vi "FGV-Funktionstasten.vi"(0 "Referenz":refnum<vi>, 1 "Samplepoint":u16, 2 "Herkunft":string="---", 5 "Funktionstasten":T4, 7 "Zeit":sgl, 9 "Zustand":T2, 11 "Fehler (FALSE)":bool, 12 "Aktion":T3=enum."Lesen") -> (3 "Samplepoint":u16, 4 "EXTERN Umschalten":bool, 6 "Zustand Herkunft AK?":bool, 8 "Zeit Zustands Anwahl":timestamp, 10 "ausgewählte Funktion":T2, 13 "Busy":bool, 14 "Betriebsart":T1, 15 "Fehler steht an":bool)   [LabVIEW 2020, in "Funktionstasten.lvlib"]
doc: "Führt die durch den Enum \"Aktion\" geforderte Aktion aus, indem über eine Referenz auf den Cluster \"Funktionstasten\" die Beschriftungen und Tastenfarben manipuliert werden. Der Eingang \"Funktionstasten\" ist neben der Referenz notwendig, um bei einer Ereignis-gesteuerten Tastenreaktion eine gedrückte Taste zui erkennen, die Latch-Verhalten hat.\n\nDie funktionale globale Variable (FGV) speichert den aktuellen Zustand der Tasten und des aktuellen Fehlerstatus. Die FGV kann von Sub-VIs und fremden VIs aufgerufen werden. Außer dem Eingang \"Aktion\" sind alle Eingänge sind nur \"empfohlen\" und nicht immer \"erforderlich\", -abhängig von der Aktion:\n\nInitialisieren:\nSpeichert eine Referenz auf den Cluster\"Funktionstasten\" und macht alle Tasten vorläufig nicht anwählbar. Erst nach dem vollständigen Hochlauf sollten die Tasten durch die Aktion \"Zustand setzen\" in einem definierten Zustand aktiviert werden. Dabei werden die Beschriftungen der Tasten vom Enum \"Zustand\" übernommen und gespeichert.\nNur Eingang \"Referenz\" erforderlich.\n\nZustand setzen:\nÄndert den Tastenzustand programmgesteuert auf den am Eingang \"Zustand\" anliegenden Wert.\nNur Eingang \"Zustand\" erforderlich.\n\nTaste gedrückt:\nMarkiert die gedrückte Taste entsprechend dem gespeicherten Fehlerzustand und liefert die ausgewählte Funktion zur Steuerung eines Zustandsautomaten.\nNur Eingang \"Funktionstasten\" erforderlich.\n\nFehler speichern:\nÜbernimmt den Eingang \"Fehler\" und speichert ihn als \"Fehler steht an\".\nNur Eingang \"Fehler\" erforderlich.\n\nZustand lesen:\nLiefert die durch den letzten Tastendruck ausgewählte, gespeicherte Funktion und den Fehlerstatus.\nKeine Eingänge notwendig.\n\nManuell:\nAktiviert den Bedienerzugriff auf die Tasten für Handbetrieb.\nKeine Eingänge notwendig.\n\nRemote:\nDie Tasten sind nur mehr über die Aktion \"Zustand setzen\" anwählbar, die aktuelle Taste und der Fehlerzustand werden aber angezeigt.\nKeine Eingänge notwendig."
uses:
  Funktionstasten.lvlib
  Funktionstasten.ctl
  Funktionstasten-Aktion.ctl
  Zustaende.ctl
  Betriebsart.ctl
  Freigabe Aktionen.ctl
  Sprachverwaltung/FGV Aktion Tabelle zerlegen.ctl
  Aktionen Zustaende Loggen.ctl
  Seiten/Anlagenuebersicht/VisBx Anzeige/Aktion FGV Ventile manuell schalten Crio.ctl
  PNS/Aktionen FGV Grenzwerte.ctl
  SysLog/SysLog Interface.ctl
  PNS/PNS.lvlib
  Sprachverwaltung/Sprachverwaltung.lvlib
  Amium PNS/Amium PNS.lvlib
  SysLog/SysLog.lvlib
  <vilib>/Utility/Data Type/NI_Data Type.lvlib
  Seiten/Anlagenuebersicht/VisBx Anzeige/Anlagenuebersicht.lvlib
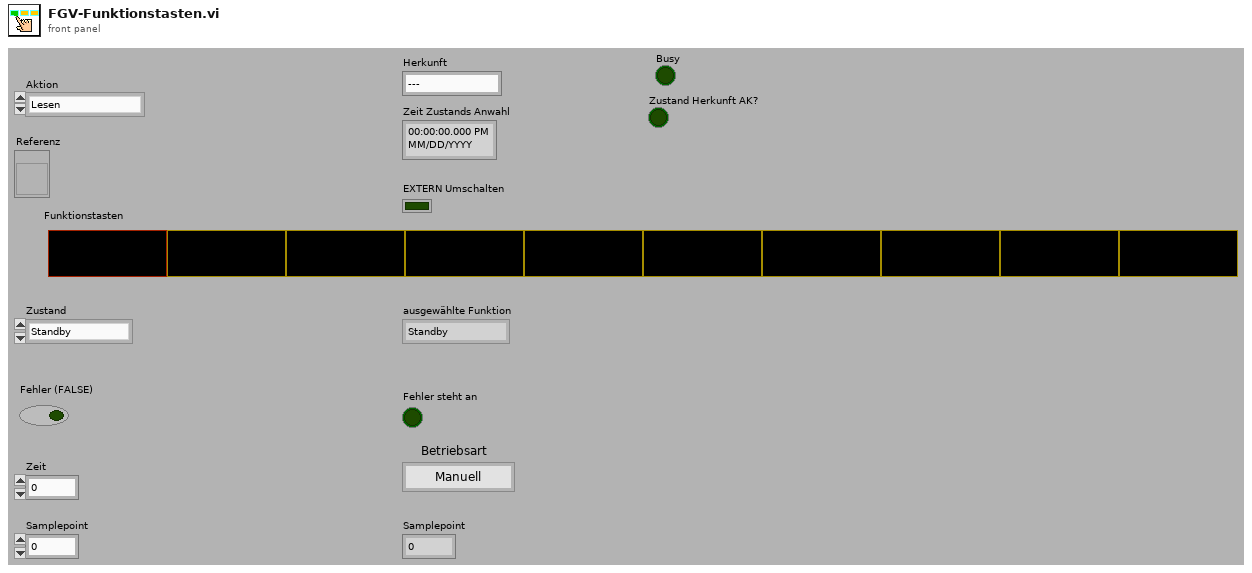
[diagram p1: front panel]
types:
  T1 = typedef "Funktionstasten.lvlib/Betriebsart.ctl" = enum16{"Manuell", "Remote", "Bitparallel"}
  T2 = typedef "Funktionstasten.lvlib/Zustaende.ctl" = enum16{"Standby", "Pause", "Eco", "Messen", "Kalibrieren", "Spülen Filter", "Spülen Leitung", "Umgebungsluft", "0-Gas", "Cal-Gas", "CG zu PNS", "-------------", "Init 1", "Init 2", "Init 3", "Init 4", "Messen vorbereiten", "Messen durchführen", "Exit"}
  T3 = typedef "Funktionstasten.lvlib/Funktionstasten-Aktion.ctl" = enum16{"Initialisieren", "Zustand setzen", "Taste gedrückt", "Fehler speichern", "Lesen", "Manuell", "Remote", "Bitparallel", "Samplepoint", "Zeit Prüfen", "reset Umschalten"}
  T4 = typedef "Funktionstasten.lvlib/Funktionstasten.ctl" = cluster{"Taste 1":bool, "Taste 2":bool, "Taste 3":bool, "Taste 4":bool, "Taste 5":bool, "Taste 6":bool, "Taste 7":bool, "Taste 11":bool, "Taste 9":bool, "Taste 10":bool}
  T5 = typedef "Funktionstasten.lvlib/Freigabe Aktionen.ctl" = enum16{"prüfen", "Freigabe?", "lesen"}
  T6 = typedef "Sprachverwaltung.lvlib/FGV Aktion Tabelle zerlegen.ctl" = enum16{"laden", "vereinzeln", "speichern"}
  T7 = typedef "Anlagenuebersicht.lvlib/Aktion FGV Ventile manuell schalten Crio.ctl" = enum16{"lesen", "Ventile schalten", "Testbetrieb aktiv", "Testbetrieb inaktiv", "Anzeige Ventilstellung"}
  T8 = typedef "Funktionstasten.lvlib/Aktionen Zustaende Loggen.ctl" = enum16{"lesen", "schreiben", "löschen", "init"}
  T9 = typedef "PNS.lvlib/Aktionen FGV Grenzwerte.ctl" = enum16{"lesen", "Grenzw. schreiben", "Anweisungscode", "IP-Adresse", "laden", "speichern", "Anweisungscode vorgeben"}
  T10 = typedef "SysLog.lvlib/SysLog Interface.ctl" = cluster{"FehlermeldungsCode":i32, "ErfolgsmeldungsCode":i32, "ParameterListenString":string, "Anzeige":bool, "SysLogIcon":enum16{"OK", "Warnung", "Fehler"}, "intern":bool}
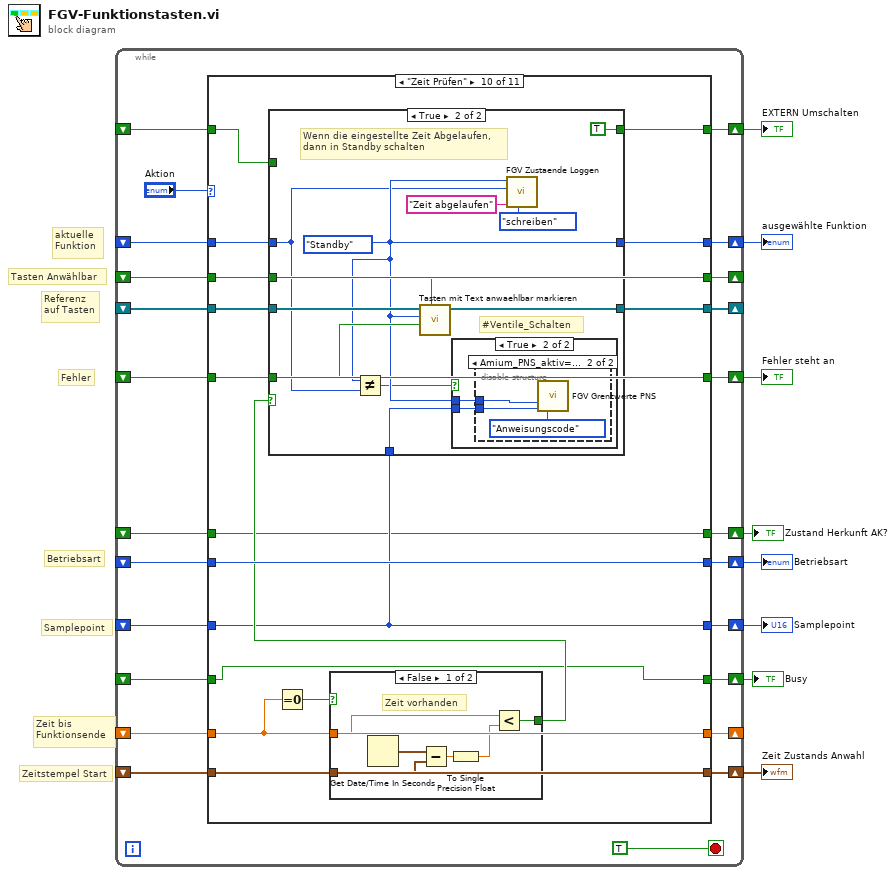
[diagram p0: block diagram]
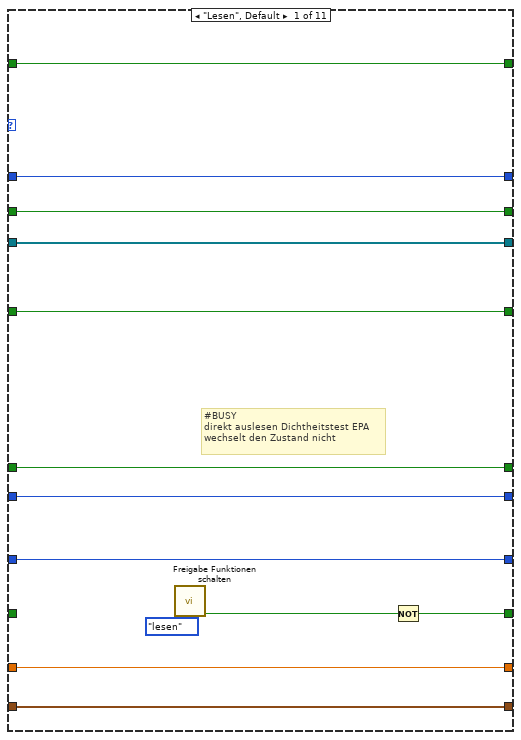
[diagram p2: hidden frame]
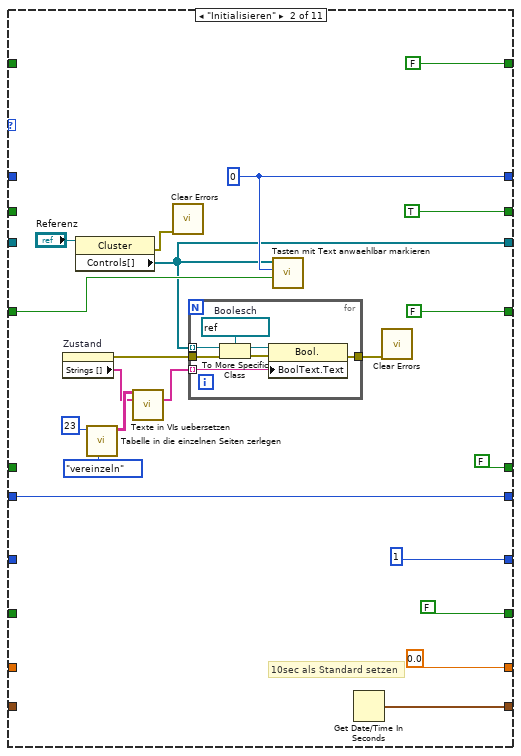
[diagram p3: hidden frame]
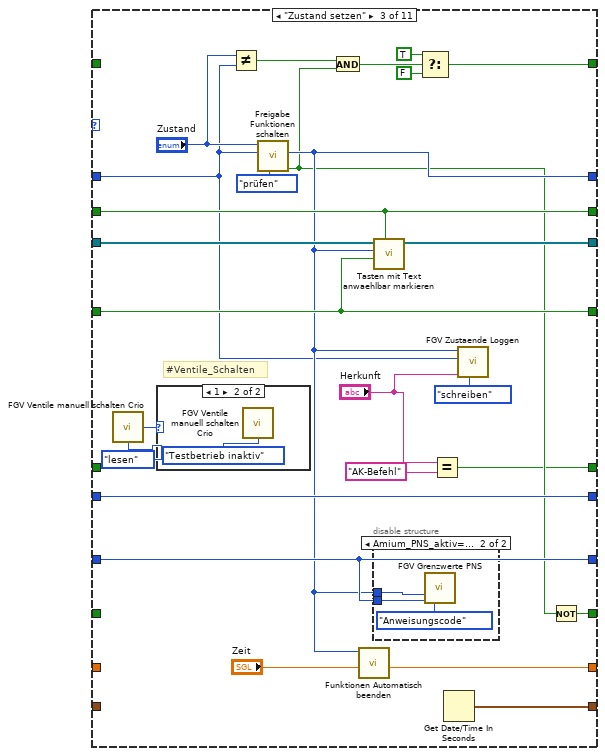
[diagram p4: hidden frame]
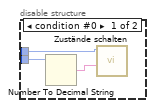
[diagram p6: hidden frame]
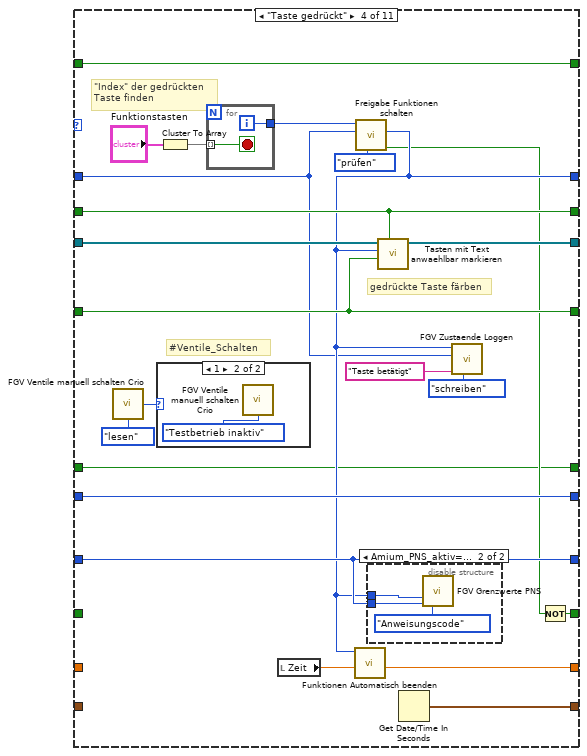
[diagram p7: hidden frame]
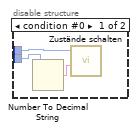
[diagram p9: hidden frame]
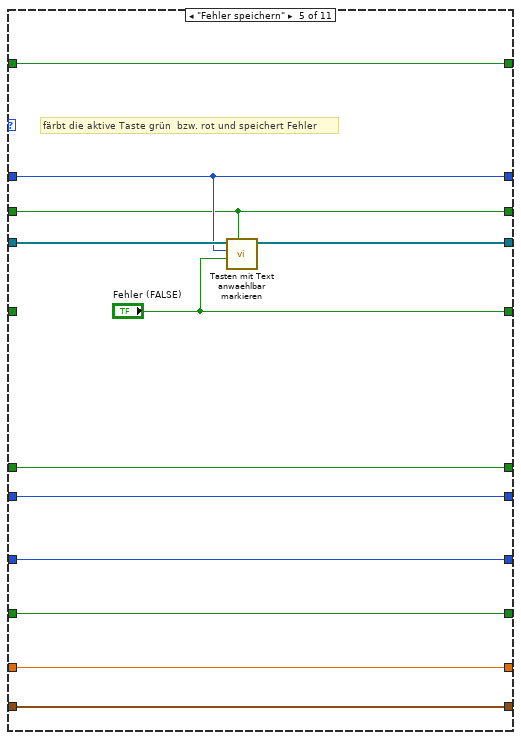
[diagram p10: hidden frame]
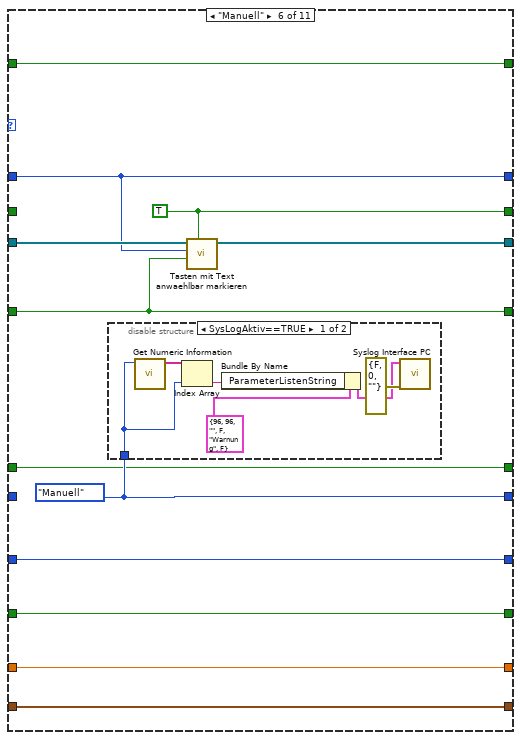
[diagram p11: hidden frame]
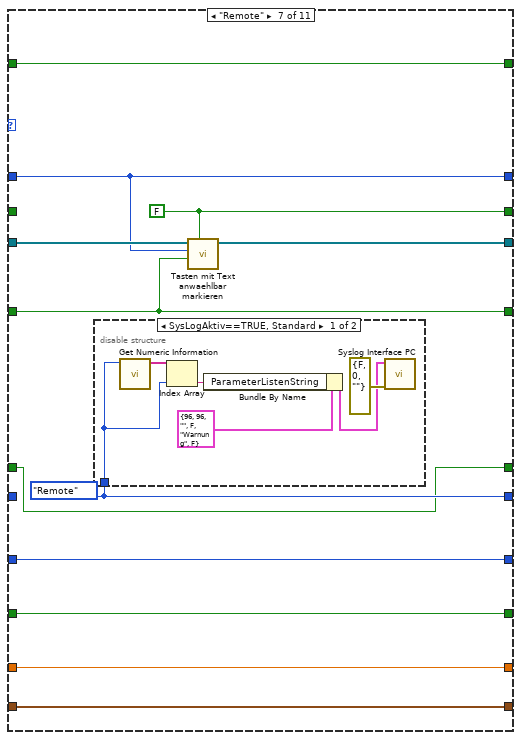
[diagram p13: hidden frame]
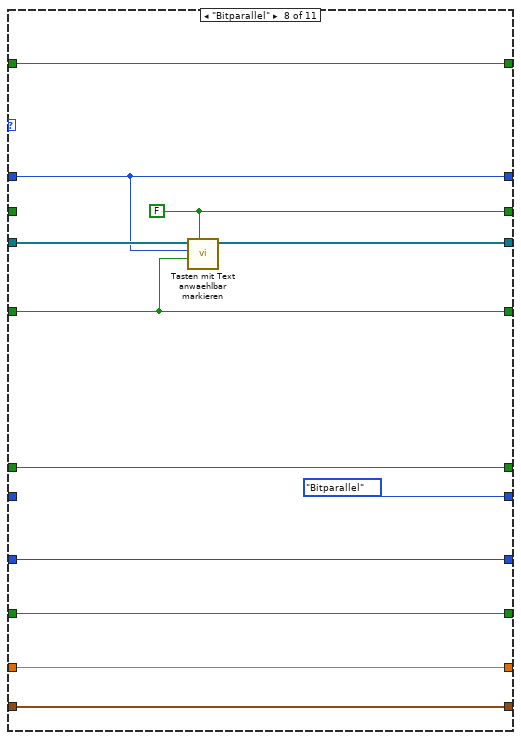
[diagram p15: hidden frame]
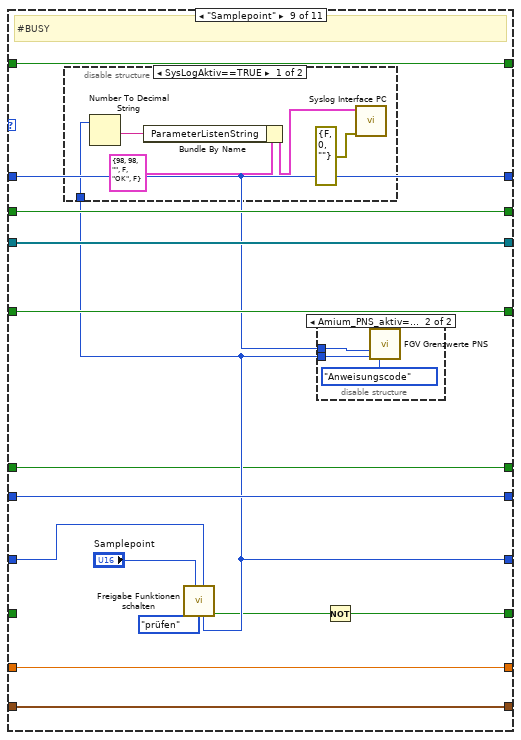
[diagram p16: hidden frame]
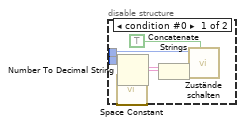
[diagram p18: hidden frame]
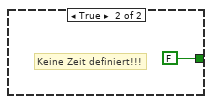
[diagram p19: hidden frame]
diagram:
  # "Zeitstempel Start"
  # "Samplepoint"
  # "Betriebsart"
  # "Tasten Anwählbar"
  # "Zeit bis \nFunktionsende"
  # "Fehler"
  # "aktuelle\nFunktion"
  # "Referenz\nauf Tasten"
  n1 = while {
    shift-right: [w18] -> w5
    shift-left: _ -> [w32]
    shift-right: [w29] -> _
    shift-left: _ -> [w28]
    shift-right: [w27] -> w8
    shift-left: _ -> [w21]
    shift-right: [w26] -> _
    shift-left: _ -> [w25]
    shift-right: [w24] -> _
    shift-left: _ -> [w23]
    shift-right: [w22] -> w7
    shift-left: _ -> [w20]
    shift-right: [w17] -> w6
    shift-left: _ -> [w19]
    shift-right: [w16] -> w3
    shift-left: _ -> [w15]
    shift-right: [w14] -> w4
    shift-left: _ -> [w13]
    shift-right: [w12] -> w2
    shift-left: _ -> [w11]
    shift-right: [w10] -> w1
    shift-left: _ -> [w9]
    stop <- TRUE stop-if-true
    n2 = case shown="\"Zeit Prüfen\"" "Aktion" {
      tunnel: w28 -> [w44 _ w99 w127 w149 w161 w177 w195 w210 w242 w279]
      tunnel: [w45 w63 w82 w114 w146 w159 w175 w193 w206 w240 w281] -> w18
      tunnel: w32 -> [w45 _ w81 w113 w146 w159 w175 w193 w206 w237 w281]
      tunnel: [w44 w62 w98 w126 w148 w160 w178 w196 w210 w239 w279] -> w29
      tunnel: w25 -> [w42 _ _ _ w150 w162 w180 w198 w211 w234 w276]
      tunnel: w21 -> [w43 w64 w96 w124 _ w157 w176 w194 w213 w241 w283]
      tunnel: [w43 FALSE ("Fehler (FALSE)") w96 w124 "Fehler (FALSE)" w157 w176 w194 w213 w241 w283] -> w27
      tunnel: [w42 sgl 0.0 w92 w121 w150 w162 w180 w198 w211 w234 w276] -> w26
      tunnel: [w41 TRUE ("Fehler (FALSE)") w97 w125 w145 w158 w179 w197 w209 w238 w280] -> w24
      tunnel: w23 -> [w41 _ w97 w125 w145 _ _ _ w209 w238 w280]
      tunnel: [w40 w60 w95 w123 w144 w153 w171 Betriebsart."Bitparallel" ("Betriebsart") w212 w243 w278] -> w22
      tunnel: w20 -> [w40 w60 w95 w123 w144 _ _ _ w212 w243 w278]
      tunnel: [w39 u16 1 ("Samplepoint") w84 w116 w143 w156 w174 w191 w202 w230 w277] -> w17
      tunnel: w19 -> [w39 _ w84 w116 w143 w156 w174 w191 w203 w230 w277]
      tunnel: [w38 w57 w94 w122 w142 w155 w173 w190 w208 w233 w275] -> w16
      tunnel: w15 -> [w38 _ _ _ w142 w155 w173 w190 w208 w233 w275]
      tunnel: [w37 FALSE w85 w117 w141 w154 w172 w189 w207 w231 FALSE] -> w14
      tunnel: w13 -> [w37 _ _ w117 w141 w154 w172 w189 w207 w232 _]
      tunnel: [w34 FALSE w80 w111 w140 w152 w170 w188 w200 w229 w274] -> w12
      tunnel: w11 -> [_ _ _ _ w140 w152 w170 w188 _ w229 w274]
      tunnel: [w36 FALSE w76 w109 w139 w151 w169 w187 w199 w228 w273] -> w10
      tunnel: w9 -> [w36 _ _ w109 w139 w151 w169 w187 w199 w228 w273]
      frame "Lesen", Default {
        # "#BUSY\ndirekt auslesen Dichtheitstest EPA \nwechselt den Zustand nicht"
        n3 = call "Freigabe Funktionen schalten.vi"("Aktionen"=Freigabe_Aktionen."lesen") -> ("Freigabe?"=w35:bool)  [unwired: 8 in, 2 out]
        n4 = Not(x=w35) -> (.not. x?=w34:bool)
      }
      frame "Initialisieren" {
        w63 = 0 ("Zustand")
        # "10sec als Standard setzen"
        n5 = property on="Zustand" class="Enum (strikt)"() -> (error out=w54:errorcluster, "Strings []"=w50:string[])  [unwired: 2 in, 1 out]
        n6 = property class="Cluster"(reference="Referenz") -> (error out=w55:errorcluster, "Controls[]"=w62:refnum<vi>[])  [unwired: 1 in, 1 out]
        n7 = call "Tabelle in die einzelnen Seiten zerlegen.vi"("Aktion"=FGV_Aktion_Tabelle_zerlegen."vereinzeln", "Index (Seite)"=23) -> ("Sprachliste"=w51:string[][])  [unwired: 7 in, 2 out]
        n8 = call "Texte in VIs uebersetzen.vi"("Sprachliste"=w51, "String-Array zum Übersetzen"=w50) -> ("String-Array zum Übersetzen"=w49:string[])  [unwired: 9 in, 4 out]
        n9 = call <vilib>:"Clear Errors.vi"("error in (no error)"=w55) -> ()  [unwired: 5 in, 2 out]
        n10 = for {
          tunnel: w49 -> [w70] mode=indexing
          tunnel: w62 -> [w72] mode=indexing
          tunnel: w54 -> [w68]
          tunnel: [w67] -> w53
          w73 = refnum<vi> refnum  # Boolesch
          n11 = To More Specific Class(target class=w73, reference=w72, error in=w68) -> (specific class reference=w71:refnum<vi>, error out=w69:errorcluster)
          n12 = property class="Bool."(reference=w71, error in=w69, "BoolText.Text"=w70) -> (error out=w67:errorcluster)  [unwired: 1 out]
        }
        n13 = call "Tasten mit Text anwaehlbar markieren.vi"("Fehler"=w64, "Tastennummer"=w63, "Tastenreferenzen"=w62) -> ()  [unwired: 2 in, 7 out]
        n14 = Get Date/Time In Seconds() -> (seconds since 1Jan1904=w57:timestamp)
        n15 = call <vilib>:"Clear Errors.vi"("error in (no error)"=w53) -> ()  [unwired: 5 in, 2 out]
      }
      frame "Zustand setzen" {
        # "#Ventile_Schalten"
        n16 = call "FGV Ventile manuell schalten Crio.vi"("Aktion"=Aktion_FGV_Ventile_manuell_schalten_Crio."lesen") -> ("Betrieb"=w75:u16)  [unwired: 11 in, 3 out]
        n17 = case shown="1" w75 {
          frame 0, Default {
          }
          frame 1 {
            n18 = call "FGV Ventile manuell schalten Crio.vi"("Aktion"=Aktion_FGV_Ventile_manuell_schalten_Crio."Testbetrieb inaktiv") -> ()  [unwired: 11 in, 4 out]
          }
        }
        n19 = Not Equal?(x="Zustand", y=w81) -> (x != y?=w89:bool)
        n20 = call "Freigabe Funktionen schalten.vi"("Aktionen"=Freigabe_Aktionen."prüfen", "Zustand ALT"=w81, "Zustand NEU"="Zustand") -> ("Freigabe?"=w79:bool, "Zustand"=w82:T2)  [unwired: 6 in, 1 out]
        n21 = And(x=w89, y=w79) -> (x .and. y?=w88:bool)
        n22 = call "Funktionen Automatisch beenden.vi"("Zeit"="Zeit", "ausgewählte Funktion"=w82) -> ("Zeit"=w92:sgl)  [unwired: 9 in]
        n23 = call "Tasten mit Text anwaehlbar markieren.vi"("Anwählbar"=w97, "Fehler"=w96, "Tastennummer"=w82, "Tastenreferenzen"=w99) -> ("Tastenreferenzen (Kopie)"=w98:refnum<vi>[])  [unwired: 2 in, 5 out]
        n24 = disable-structure shown="Amium_PNS_aktiv==FALSE" {
          disable-tunnel: w84 -> [w101 w105]
          disable-tunnel: w82 -> [w103 w104]
          frame condition #0 {
            n25 = Number To Decimal String(number=w101) -> (decimal integer string=w102:string)  [unwired: 1 in]
            n26 = call "Zustände schalten.vi"("Samplepoint 2"=w102, "Zustand"=w103) -> ()  [unwired: 9 in, 1 out]
          }
          frame condition #1 (active) {
            n27 = call "FGV Grenzwerte PNS.vi"("Zustand"=w104, "Samplepoint"=w105, "Aktionen FGV Grenzwerte"=Aktionen_FGV_Grenzwerte."Anweisungscode") -> ()  [unwired: 10 in, 3 out]
          }
        }
        n28 = Select(t=TRUE, s=w88, f=FALSE) -> (s? t:f=w85:bool)
        n29 = Equal?(x="Herkunft", y="AK-Befehl" ("Herkunft")) -> (x = y?=w76:bool)
        n30 = Get Date/Time In Seconds() -> (seconds since 1Jan1904=w94:timestamp)
        n31 = call "FGV Zustaende Loggen.vi"("Aktionen Zustände Loggen"=Aktionen_Zustaende_Loggen."schreiben", "Herkunft"="Herkunft", "Zustand ALT"=w81, "Zustand NEU"=w82) -> ()  [unwired: 6 in, 2 out]
        n32 = Not(x=w79) -> (.not. x?=w80:bool)
      }
      frame "Taste gedrückt" {
        # "#Ventile_Schalten"
        # "gedrückte Taste färben"
        # "\"Index\" der gedrückten\nTaste finden"
        n33 = call "FGV Ventile manuell schalten Crio.vi"("Aktion"=Aktion_FGV_Ventile_manuell_schalten_Crio."lesen") -> ("Betrieb"=w107:u16)  [unwired: 11 in, 3 out]
        n34 = case shown="1" w107 {
          frame 0, Default {
          }
          frame 1 {
            n35 = call "FGV Ventile manuell schalten Crio.vi"("Aktion"=Aktion_FGV_Ventile_manuell_schalten_Crio."Testbetrieb inaktiv") -> ()  [unwired: 11 in, 4 out]
          }
        }
        n36 = Cluster To Array(cluster="Funktionstasten") -> (array=w129:bool[])
        n37 = for {
          tunnel: w129 -> [w137] mode=indexing
          tunnel: [w138] -> w119
          i -> [w138]
          stop <- w137 stop-if-true
        }
        n38 = local read "Zeit"() -> (w118:sgl)
        n39 = call "Freigabe Funktionen schalten.vi"("Aktionen"=Freigabe_Aktionen."prüfen", "Zustand ALT"=w113, "Zustand NEU"=w119) -> ("Freigabe?"=w110:bool, "Zustand"=w114:T2)  [unwired: 6 in, 1 out]
        n40 = call "Funktionen Automatisch beenden.vi"("Zeit"=w118, "ausgewählte Funktion"=w114) -> ("Zeit"=w121:sgl)  [unwired: 9 in]
        n41 = disable-structure shown="Amium_PNS_aktiv==FALSE" {
          disable-tunnel: w116 -> [w132 w135]
          disable-tunnel: w114 -> [w133 w134]
          frame condition #0 {
            n42 = Number To Decimal String(number=w132) -> (decimal integer string=w131:string)  [unwired: 1 in]
            n43 = call "Zustände schalten.vi"("Samplepoint 2"=w131, "Zustand"=w133) -> ()  [unwired: 9 in, 1 out]
          }
          frame condition #1 (active) {
            n44 = call "FGV Grenzwerte PNS.vi"("Zustand"=w134, "Samplepoint"=w135, "Aktionen FGV Grenzwerte"=Aktionen_FGV_Grenzwerte."Anweisungscode") -> ()  [unwired: 10 in, 3 out]
          }
        }
        n45 = call "Tasten mit Text anwaehlbar markieren.vi"("Anwählbar"=w125, "Fehler"=w124, "Tastennummer"=w114, "Tastenreferenzen"=w127) -> ("Tastenreferenzen (Kopie)"=w126:refnum<vi>[])  [unwired: 1 in, 6 out]
        n46 = Get Date/Time In Seconds() -> (seconds since 1Jan1904=w122:timestamp)
        n47 = call "FGV Zustaende Loggen.vi"("Aktionen Zustände Loggen"=Aktionen_Zustaende_Loggen."schreiben", "Herkunft"="Taste betätigt", "Zustand ALT"=w113, "Zustand NEU"=w114) -> ()  [unwired: 6 in, 2 out]
        n48 = Not(x=w110) -> (.not. x?=w111:bool)
      }
      frame "Fehler speichern" {
        # "färbt die aktive Taste grün  bzw. rot und speichert Fehler"
        n49 = call "Tasten mit Text anwaehlbar markieren.vi"("Anwählbar"=w145, "Fehler"="Fehler (FALSE)", "Tastennummer"=w146, "Tastenreferenzen"=w149) -> ("Tastenreferenzen (Kopie)"=w148:refnum<vi>[])  [unwired: 1 in, 6 out]
      }
      frame "Manuell" {
        w153 = Betriebsart."Manuell" ("Betriebsart")
        w158 = TRUE ("Anwählbar")
        n50 = disable-structure shown="SysLogAktiv==TRUE" {
          disable-tunnel: w153 -> [w166 _]
          frame condition #0 (active) {
            n51 = call <vilib>:"Get Numeric Information.vi"("variant"=w166) -> ("enum names"=w167:string[])  [unwired: 7 in, 3 out]
            n52 = Index Array(array=w167, index=w166) -> (element=w163:string)
            n53 = Bundle By Name(cluster=T10 {"FehlermeldungsCode"=96, "ErfolgsmeldungsCode"=96, "ParameterListenString"="", "Anzeige"=FALSE, "SysLogIcon"=enum."Warnung", "intern"=FALSE} ("Cluster (in)"), "ParameterListenString"=w163) -> (w164:T10)
            n54 = call "Syslog Interface PC.vi"("Fehler (in)"=errorcluster {"status"=FALSE, "code"=0, "source"=""}, "Cluster (in)"=w164) -> ()  [unwired: 9 in, 1 out]
          }
          frame condition #1 {
          }
        }
        n55 = call "Tasten mit Text anwaehlbar markieren.vi"("Anwählbar"=w158, "Fehler"=w157, "Tastennummer"=w159, "Tastenreferenzen"=w161) -> ("Tastenreferenzen (Kopie)"=w160:refnum<vi>[])  [unwired: 1 in, 6 out]
      }
      frame "Remote" {
        w171 = Betriebsart."Remote" ("Betriebsart")
        w179 = FALSE ("Anwählbar")
        n56 = disable-structure shown="SysLogAktiv==TRUE, Standard" {
          disable-tunnel: w171 -> [w184 _]
          frame condition #0 (active) {
            n57 = call <vilib>:"Get Numeric Information.vi"("variant"=w184) -> ("enum names"=w185:string[])  [unwired: 7 in, 3 out]
            n58 = Index Array(array=w185, index=w184) -> (element=w181:string)
            n59 = Bundle By Name(cluster=T10 {"FehlermeldungsCode"=96, "ErfolgsmeldungsCode"=96, "ParameterListenString"="", "Anzeige"=FALSE, "SysLogIcon"=enum."Warnung", "intern"=FALSE} ("Cluster (in)"), "ParameterListenString"=w181) -> (w182:T10)
            n60 = call "Syslog Interface PC.vi"("Fehler (in)"=errorcluster {"status"=FALSE, "code"=0, "source"=""}, "Cluster (in)"=w182) -> ()  [unwired: 9 in, 1 out]
          }
          frame condition #1 {
          }
        }
        n61 = call "Tasten mit Text anwaehlbar markieren.vi"("Anwählbar"=w179, "Fehler"=w176, "Tastennummer"=w175, "Tastenreferenzen"=w177) -> ("Tastenreferenzen (Kopie)"=w178:refnum<vi>[])  [unwired: 1 in, 6 out]
      }
      frame "Bitparallel" {
        w197 = FALSE ("Anwählbar")
        n62 = call "Tasten mit Text anwaehlbar markieren.vi"("Anwählbar"=w197, "Fehler"=w194, "Tastennummer"=w193, "Tastenreferenzen"=w195) -> ("Tastenreferenzen (Kopie)"=w196:refnum<vi>[])  [unwired: 1 in, 6 out]
      }
      frame "Samplepoint" {
        # "#BUSY"
        n63 = call "Freigabe Funktionen schalten.vi"("Samplepoint ALT"=w203, "Aktionen"=Freigabe_Aktionen."prüfen", "Samplepoint NEU"="Samplepoint") -> ("Freigabe?"=w201:bool, "Samplepoint"=w202:u16)  [unwired: 6 in, 1 out]
        n64 = disable-structure shown="SysLogAktiv==TRUE" {
          disable-tunnel: w202 -> [w217 _]
          frame condition #0 (active) {
            n65 = Number To Decimal String(number=w217) -> (decimal integer string=w214:string)  [unwired: 1 in]
            n66 = Bundle By Name(cluster=T10 {"FehlermeldungsCode"=98, "ErfolgsmeldungsCode"=98, "ParameterListenString"="", "Anzeige"=FALSE, "SysLogIcon"=enum."OK", "intern"=FALSE} ("Cluster (in)"), "ParameterListenString"=w214) -> (w215:T10)
            n67 = call "Syslog Interface PC.vi"("Fehler (in)"=errorcluster {"status"=FALSE, "code"=0, "source"=""}, "Cluster (in)"=w215) -> ()  [unwired: 9 in, 1 out]
          }
          frame condition #1 {
          }
        }
        n68 = disable-structure shown="Amium_PNS_aktiv==FALSE, Standard" {
          disable-tunnel: w206 -> [w224 w226]
          disable-tunnel: w202 -> [w221 w225]
          frame condition #0 {
            n69 = call <vilib>:"Space Constant.vi"() -> ("String"=w219:string)
            n70 = Number To Decimal String(number=w221) -> (decimal integer string=w222:string)  [unwired: 1 in]
            n71 = Concatenate Strings(w219, w222) -> (w220:string)
            n72 = call "Zustände schalten.vi"("Samplepoint setzen"=TRUE, "Samplepoint 2"=w220, "Zustand"=w224) -> ()  [unwired: 8 in, 1 out]
          }
          frame condition #1 (active) {
            n73 = call "FGV Grenzwerte PNS.vi"("Zustand"=w226, "Samplepoint"=w225, "Aktionen FGV Grenzwerte"=Aktionen_FGV_Grenzwerte."Anweisungscode") -> ()  [unwired: 10 in, 3 out]
          }
        }
        n74 = Not(x=w201) -> (.not. x?=w200:bool)
      }
      frame "Zeit Prüfen" {
        n75 = Equal To 0?(x=w234) -> (x = 0?=w235:bool)
        n76 = case shown="False" w235 {
          tunnel: w233 -> [w249 _]
          tunnel: [w245 FALSE] -> w236
          tunnel: w234 -> [w244 _]
          frame False {
            # "Zeit vorhanden"
            n77 = Get Date/Time In Seconds() -> (seconds since 1Jan1904=w248:timestamp)
            n78 = Subtract(x=w248, y=w249) -> (x-y=w247:dbl)
            n79 = To Single Precision Float(number=w247) -> (single precision float=w246:sgl)
            n80 = Less?(x=w244, y=w246) -> (x < y?=w245:bool)
          }
          frame True {
            # "Keine Zeit definiert!!!"
          }
        }
        n81 = case shown="True" w236 {
          tunnel: w242 -> [w252 w264]
          tunnel: w241 -> [_ w263]
          tunnel: [w253 w256] -> w240
          tunnel: [w252 w262] -> w239
          tunnel: w238 -> [_ w261]
          tunnel: w237 -> [w253 w255]
          tunnel: w232 -> [w251 _]
          tunnel: [w251 TRUE] -> w231
          tunnel: w230 -> [_ w259]
          frame False {
          }
          frame True {
            w256 = Zustaende."Standby" ("Zustand")
            # "#Ventile_Schalten"
            # "Wenn die eingestellte Zeit Abgelaufen,\ndann in Standby schalten"
            n82 = Not Equal?(x=w256, y=w255) -> (x != y?=w254:bool)
            n83 = call "Tasten mit Text anwaehlbar markieren.vi"("Anwählbar"=w261, "Fehler"=w263, "Tastennummer"=w256, "Tastenreferenzen"=w264) -> ("Tastenreferenzen (Kopie)"=w262:refnum<vi>[])  [unwired: 2 in, 5 out]
            n84 = case shown="True" w254 {
              tunnel: w259 -> [_ w266]
              tunnel: w256 -> [_ w265]
              frame False {
              }
              frame True {
                n85 = disable-structure shown="Amium_PNS_aktiv==FALSE" {
                  disable-tunnel: w266 -> [w268 w271]
                  disable-tunnel: w265 -> [w269 w270]
                  frame condition #0 {
                    n86 = Number To Decimal String(number=w268) -> (decimal integer string=w267:string)  [unwired: 1 in]
                    n87 = call "Zustände schalten.vi"("Samplepoint 2"=w267, "Zustand"=w269) -> ()  [unwired: 9 in, 1 out]
                  }
                  frame condition #1 (active) {
                    n88 = call "FGV Grenzwerte PNS.vi"("Zustand"=w270, "Samplepoint"=w271, "Aktionen FGV Grenzwerte"=Aktionen_FGV_Grenzwerte."Anweisungscode") -> ()  [unwired: 10 in, 3 out]
                  }
                }
              }
            }
            n89 = call "FGV Zustaende Loggen.vi"("Aktionen Zustände Loggen"=Aktionen_Zustaende_Loggen."schreiben", "Herkunft"="Zeit abgelaufen", "Zustand ALT"=w255, "Zustand NEU"=w256) -> ()  [unwired: 6 in, 2 out]
          }
        }
      }
      frame "reset Umschalten" {
      }
    }
  }
  "Fehler steht an" <- w8
  "ausgewählte Funktion" <- w5
  "Betriebsart" <- w7
  "Samplepoint" <- w6
  "EXTERN Umschalten" <- w4
  "Zeit Zustands Anwahl" <- w3
  "Busy" <- w2
  "Zustand Herkunft AK?" <- w1
